vi "SDSU_MemoryRestore.vi"(7 "arg":string, 8 "address":string, 9 "type":string, 10 "board":i16, 11 "refnum":i32) -> (0 "error out":errorcluster, 3 "refnum out":i32)   [LabVIEW 2016]
panel:
  in  "error in (no error)":errorcluster
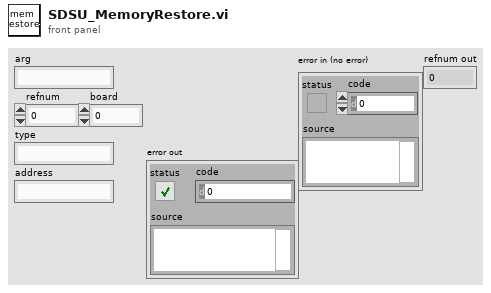
[diagram p1: front panel]
types:
  T1 = typedef "SDSU_MemLoc.ctl" = cluster{"board":i32, "type":string, "address":i32, "value":u32}
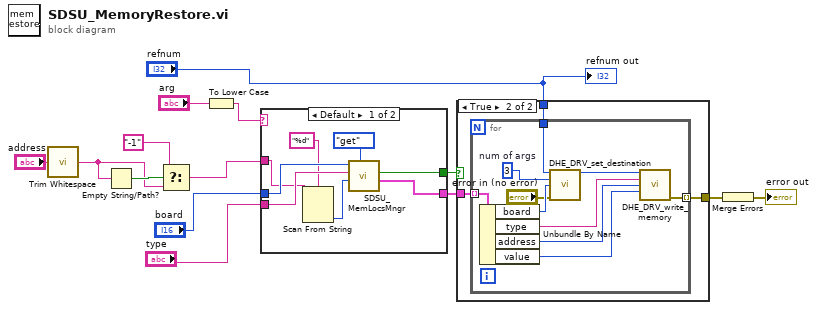
[diagram p0: block diagram]
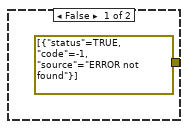
[diagram p2: hidden frame]
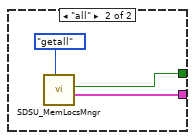
[diagram p3: hidden frame]
diagram:
  n1 = call <vilib>:"Trim Whitespace.vi"("string"="address") -> ("trimmed string"=w3:string)  [unwired: 1 in]
  n2 = Empty String/Path?(string/path=w3) -> (empty?=w4:bool)
  n3 = Select(t="-1", s=w4, f=w3) -> (s? t:f=w2:string)
  n4 = To Lower Case(string="arg") -> (all lower case string=w14:string)
  n5 = case shown="Default" w14 {
    tunnel: [w19 w24] -> w13
    tunnel: "board" -> [w21 _]
    tunnel: "type" -> [w20 _]
    tunnel: [w18 w23] -> w12
    tunnel: w2 -> [w17 _]
    frame Default {
      n6 = Scan From String(format string="%d", input string=w17) -> (output 1=w15:i32)  [unwired: 3 in, 3 out]
      n7 = call "SDSU_MemLocsMngr.vi"("action"=enum16{"set", "get", "clear", "getall"}."get", "address"=w15, "type"=w20, "board"=w21) -> ("array"=w19:T1[], "found"=w18:bool)  [unwired: 6 in]
    }
    frame "all" {
      n8 = call "SDSU_MemLocsMngr.vi"("action"=enum16{"set", "get", "clear", "getall"}."getall") -> ("array"=w24:T1[], "found"=w23:bool)  [unwired: 9 in]
    }
  }
  n9 = case shown="True" w12 {
    tunnel: w13 -> [_ w29]
    tunnel: [errorcluster[] [{"status"=TRUE, "code"=-1, "source"="ERROR not found"}] w28] -> w6
    tunnel: "refnum" -> [_ w27]
    frame False {
    }
    frame True {
      n10 = for {
        tunnel: w29 -> [w36] mode=indexing
        tunnel: w27 -> [w37]
        tunnel: [w35] -> w28 mode=indexing
        w39 = 3  # num of args
        n11 = Unbundle By Name(w36) -> ("board"=w34:i32, "type"=w33:string, "address"=w32:i32, "value"=w31:u32)
        n12 = call "DHE_DRV_set_destination.vi"("fd"=w37, "num of args"=w39, "board dest"=w34, "error in (no error)"="error in (no error)") -> ("fd out"=w38:i32)  [unwired: 11 out]
        n13 = call "DHE_DRV_write_memory.vi"("fd"=w38, "type"=w33, "address"=w32, "value"=w31) -> ("error out"=w35:errorcluster)  [unwired: 1 in, 10 out]
      }
    }
  }
  n14 = Merge Errors(w6) -> (→"error out":errorcluster)
  "refnum out" <- "refnum"
